vi "ABR-Read Data.vi"(0 "Path":path, 11 "error in (no error)":errorcluster) -> (4 "Header":T1, 6 "Neural":dbl[][](array[numeric]), 8 "CM":dbl[][](array[numeric]), 10 "I-O":dbl[][](array[numeric]), 14 "Analysis":T2, 15 "error out":errorcluster)   [LabVIEW 2020]
uses:
  TypeDefs/ABR-Analysis State.ctl
  Threshold Estimation VIs/ABR3-Threshold Estimation Result.ctl
  TypeDefs/ABR-Data Header.ctl
  epl-vi-lib/Utility VIs/Array Manipulation VIs/Array-Dimensions (2D).vi
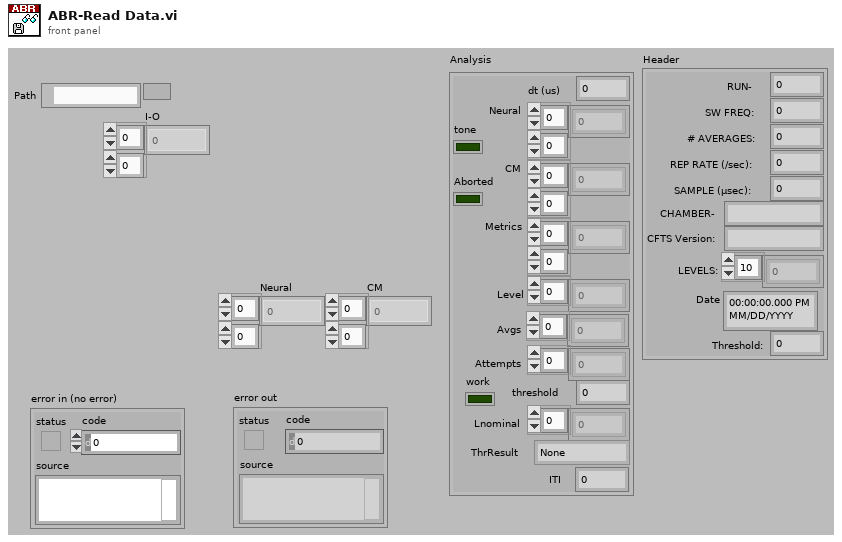
[diagram p1: front panel]
types:
  T1 = typedef "ABR-Data Header.ctl" = cluster{"RUN-":i32, "SW FREQ:":dbl, "# AVERAGES:":i32, "REP RATE (/sec):":dbl, "SAMPLE (µsec):":dbl, "CHAMBER-":string, "CFTS Version: ":string, "LEVELS:":dbl[], "Date":timestamp, "Threshold:":dbl}
  T2 = typedef "ABR-Analysis State.ctl" = cluster{"dt (us)":dbl, "Neural":dbl[][], "CM":dbl[][], "Metrics":dbl[][], "Level":dbl[], "Avgs":i32[], "Attempts":i32[], "Aborted":bool, "threshold":dbl, "Lnominal":dbl[], "tone":bool, "work":bool, "ThrResult":T3, "ITI":dbl}
  T3 = typedef "ABR3-Threshold Estimation Result.ctl" = enum16{"None", "Power", "Sigmoid", "Power (noisy)", "Suprathreshold", "Invalid"}
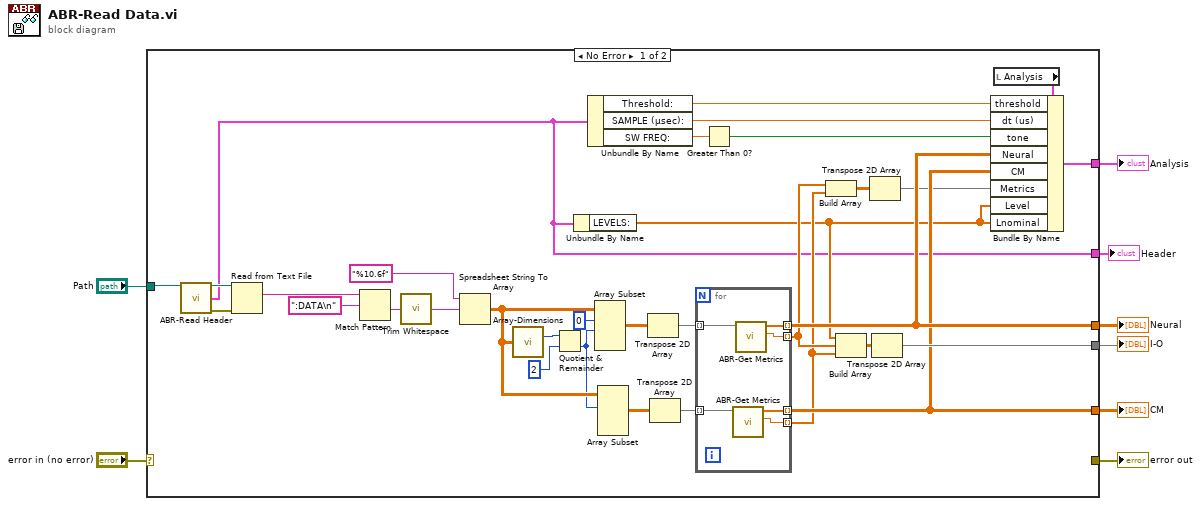
[diagram p0: block diagram]
diagram:
  n1 = case shown="No Error" "error in (no error)" {
    selector: "error in (no error)" -> [_ w48]
    tunnel: [_ w48] -> w7
    tunnel: "Path" -> [w12 _]
    tunnel: [w23 _] -> w5
    tunnel: [w22 _] -> w4
    tunnel: [w27 _] -> w3
    tunnel: [w24 _] -> w2
    tunnel: [w9 _] -> w1
    frame No Error {
      n2 = call "ABR-Read Header.vi"("Path"=w12) -> ("Path (thru)"=w13:path, "Header"=w9:T1, "error out"=w14:errorcluster)  [unwired: 12 in]
      n3 = Read from Text File(file (use dialog)=w13, error in=w14) -> (text=w41:string)  [unwired: 2 in, 3 out]
      n4 = Match Pattern(string=w41, regular expression=":DATA\n" ("search string/char (-)")) -> (after substring=w32:string)  [unwired: 1 in, 3 out]
      n5 = call <vilib>:"Trim Whitespace.vi"("string"=w32) -> ("trimmed string"=w10:string)  [unwired: 1 in]
      n6 = Spreadsheet String To Array(format string="%10.6f" ("spreadsheet string"), spreadsheet string=w10) -> (array=w35:dbl[][])  [unwired: 2 in]
      n7 = call-poly "Array-Dimensions.vi"("2D Array"=w35) -> ("# rows"=w39:i32)  [unwired: 13 in, 1 out]
      n8 = Quotient & Remainder(x=w39, y=2) -> (floor(x/y)=w33:i32)  [unwired: 1 out]
      n9 = Unbundle By Name(w9) -> ("LEVELS:"=w17:dbl[])
      n10 = Unbundle By Name(w9) -> ("Threshold:"=w11:dbl, "SAMPLE (µsec):"=w26:dbl, "SW FREQ:"=w16:dbl)
      n11 = Array Subset(array=w35, index (row)=0 ("index"), length (row)=w33) -> (w36:dbl[][])  [unwired: 2 in]
      n12 = Array Subset(array=w35, index (row)=w33) -> (w34:dbl[][])  [unwired: 3 in]
      n13 = Transpose 2D Array(2D array=w36) -> (transposed array=w30:dbl[][])
      n14 = Transpose 2D Array(2D array=w34) -> (transposed array=w29:dbl[][])
      n15 = for {
        tunnel: w30 -> [w43] mode=indexing
        tunnel: w29 -> [w42] mode=indexing
        tunnel: [w47] -> w23 mode=indexing
        tunnel: [w46] -> w22 mode=indexing
        tunnel: [w45] -> w19 mode=indexing
        tunnel: [w44] -> w18 mode=indexing
        n16 = call "ABR-Get Metrics.vi"("Data in"=w42) -> ("spread value"=w44:dbl, "Data out"=w46:dbl[])  [unwired: 8 in, 1 out]
        n17 = call "ABR-Get Metrics.vi"("Data in"=w43) -> ("spread value"=w45:dbl, "Data out"=w47:dbl[])  [unwired: 8 in, 1 out]
      }
      n18 = Greater Than 0?(x=w16) -> (x > 0?=w15:bool)
      n19 = Build Array(w19, w18) -> (w21:dbl[][])
      n20 = Build Array(w17, w19, w18) -> (w28:dbl[][])
      n21 = Transpose 2D Array(2D array=w21) -> (transposed array=w20:dbl[][])
      n22 = Transpose 2D Array(2D array=w28) -> (transposed array=w27:dbl[][])
      n23 = local read "Analysis"() -> (w25:T2)
      n24 = Bundle By Name(cluster=w25, "threshold"=w11, "dt (us)"=w26, "tone"=w15, "Neural"=w23, "CM"=w22, "Metrics"=w20, "Level"=w17, "Lnominal"=w17) -> (w24:T2)
    }
    frame Error {
    }
  }
  "error out" <- w7
  "Neural" <- w5
  "CM" <- w4
  "I-O" <- w3
  "Analysis" <- w2
  "Header" <- w1
